vi "User Events copy.vi"() -> ()   [LabVIEW 2019]
uses:
  <vilib>/event_ctls.llb/lveventtype.ctl
  <vilib>/Utility/miscctls.llb/LVTextColorsTypeDef.ctl
panel:
  out "Numero":i32
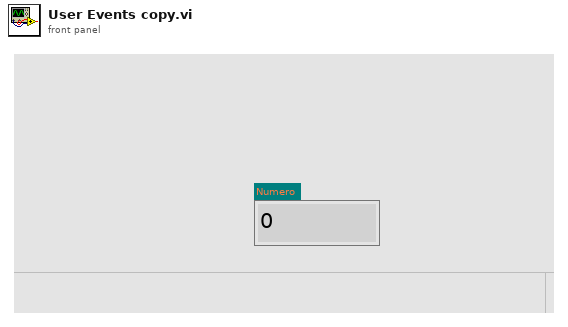
[diagram p1: front panel]
types:
  T1 = typedef "lveventtype.ctl" = enum32{"Null", "Timeout", "Annotation Menu Selection", "Annotation Menu Selection?", "App Instance Close", "App Instance Close?", "Autoscale Range Change", "Bookmark Info Change", "Cell Edit", "Cell Edit?", "Cursor Grab", "Cursor Grab?", "Cursor Menu Selection", "Cursor Menu Selection?", "Cursor Move", "Cursor Release", "Data Change", "Direction Change", "Display State Change", "Drag Ended", "Drag Enter", "Drag Leave", "Drag Over", "Drag Source Update", "Drag Starting", "Drag Starting?", "Drop", "Exec State Change", "Key Down", "Key Down?", "Key Repeat", "Key Repeat?", "Key Up", "Listbox Double Click", "Menu Activation?", "Menu Selection (App)", "Menu Selection? (App)", "Menu Selection (User)", "Mouse Down", "Mouse Down?", "Mouse Enter", "Mouse Leave", "Mouse Move", "Mouse Up", "Mouse Wheel", "NI Security User Change (App)", "Pane Size", "Panel Close", "Panel Close?", "Panel Resize", "Plot Attribute Change", "Scale Range Change", "Shortcut Menu Activation?", "Shortcut Menu Selection (App)", "Shortcut Menu Selection? (App)", "Shortcut Menu Selection (User)", "Tree Double Click", "Tree Drag", "Tree Drag?", "Tree Drop", "Tree Drop?", "Tree Item Close", "Tree Item Close?", "Tree Item Open", "Tree Item Open?", "User Event", "Value Change"}
  T2 = typedef "LVTextColorsTypeDef.ctl" = cluster{"Text Color":u32, "Background Color":u32}
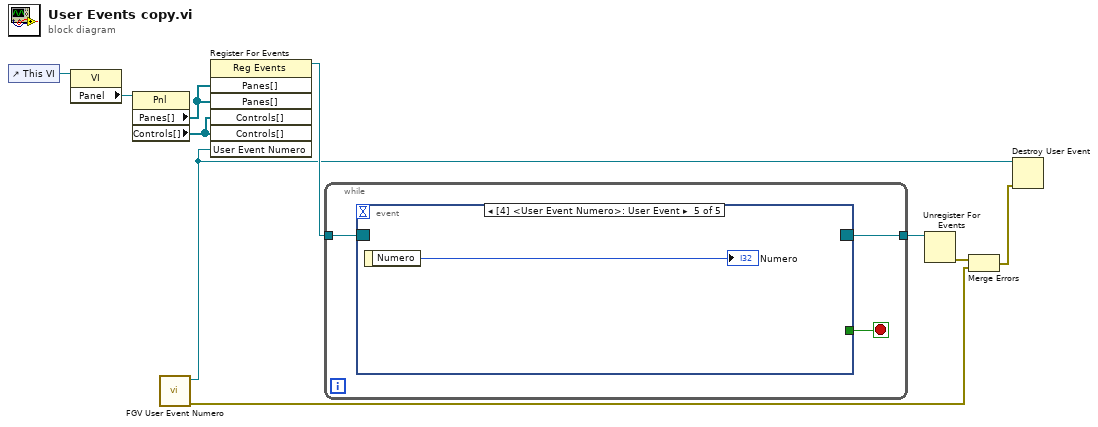
[diagram p0: block diagram]
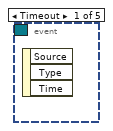
[diagram p2: hidden frame]
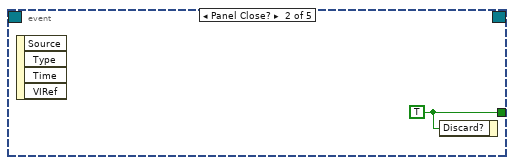
[diagram p3: hidden frame]
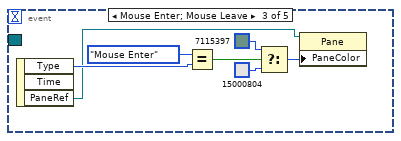
[diagram p4: hidden frame]
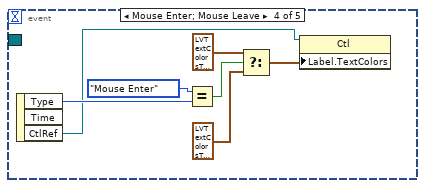
[diagram p5: hidden frame]
diagram:
  n1 = control-ref of="This VI"() -> (w5:refnum<vi>)
  n2 = property class="VI"(reference=w5) -> ("Panel"=w3:refnum<vi>)  [unwired: 1 in, 2 out]
  n3 = property class="Pnl"(reference=w3) -> ("Panes[]"=w4:refnum<vi>[], "Controls[]"=w2:refnum<vi>[])  [unwired: 1 in, 2 out]
  n4 = call "FGV User Event Numero.vi"() -> ("error out"=w10:errorcluster, "User Event Numero"=w1:refnum<user-event>)  [unwired: 10 in]
  n5 = register-events(w4, w4, w2, w2, w1) -> (reference out=w7:refnum<event-registration>)  [unwired: 2 in, 1 out]
  n6 = while {
    tunnel: w7 -> [w12]
    tunnel: [w11] -> w6
    stop <- w13 stop-if-true
    n7 = event shown="[4] <User Event Numero>: User Event" {
      selector: w12 -> [_ _ _ _ _]
      dyn-events: [_ _ _ _ _] -> w11
      timeout: _ -> [_ _ _ _ _]
      tunnel: [_ w14 _ _ _] -> w13
      event Timeout {
        n8 = event-data() -> ()  [unwired: 1 in, 3 out]
      }
      event Panel Close? {
        w14 = TRUE ("Discard?")
        n9 = event-data() -> ()  [unwired: 1 in, 4 out]
        n10 = event-data("Discard?"=w14) -> ()  [unwired: 1 in, 1 out]
      }
      event Mouse Enter; Mouse Leave {
        n11 = event-data() -> ("Type"=w21:T1, "PaneRef"=w15:refnum<vi>)  [unwired: 1 in, 1 out]
        n12 = Equal?(x=lveventtype."Mouse Enter", y=w21) -> (x = y?=w19:bool)
        n13 = Select(t=u32 7115397, s=w19, f=u32 15000804) -> (s? t:f=w18:u32)
        n14 = property class="Pane"(reference=w15, "PaneColor"=w18) -> ()  [unwired: 1 in, 2 out]
      }
      event Mouse Enter; Mouse Leave {
        n15 = event-data() -> ("Type"=w28:T1, "CtlRef"=w25:refnum<vi>)  [unwired: 1 in, 1 out]
        n16 = Equal?(x=lveventtype."Mouse Enter", y=w28) -> (x = y?=w26:bool)
        n17 = Select(t=T2 {"Text Color"=16250871, "Background Color"=11522989} ("Label.Text Colors"), s=w26, f=T2 {"Text Color"=16743234, "Background Color"=32639} ("Label.Text Colors")) -> (s? t:f=w23:T2)
        n18 = property class="Ctl"(reference=w25, "Label.TextColors"=w23) -> ()  [unwired: 1 in, 2 out]
      }
      event User Event {
        n19 = event-data() -> ("Numero"=→"Numero":i32)  [unwired: 1 in]
      }
    }
  }
  n20 = Unregister For Events(event registration refnum=w6) -> (error out=w8:errorcluster)  [unwired: 1 in]
  n21 = Merge Errors(w8, w10) -> (w9:errorcluster)
  n22 = Destroy User Event(user event=w1, error in=w9) -> ()  [unwired: 1 out]
